vi "OSA_example.vi"() -> ()   [LabVIEW 2010]
doc: "Example GUI for continous or single asyncronous acquisition and plotting of interferogram and spectrum with datareduction. \n\nWhen creating custom dataacquisition applications displaying data; copy the graphs in this example, create corresponding graph references and connect to the init vi, see example diagram.\n\nRoutines with white icon background can be found in the TREE vi.\nRoutines with yellow icon background are specific for this example.\n\nMake sure there is no duplicate of FTSLV.dll, as otherwise FTSLib.dll and the Labview drivers might not be accessing the same library."
uses:
  _OSA_class/OSA.lvclass
  _OSA_class/typeDef/queue_action.ctl
  _OSA_class/typeDef/acq_dataType.ctl
  _OSA_class/typeDef/apodisation.ctl
  _OSA_class/misc_examples/ctrlRefs.ctl
  _OSA_class/misc_examples/action_data.ctl
  _OSA_class/typeDef/PDTemperatureMode.ctl
  _OSA_class/typeDef/resolution.ctl
  _OSA_class/typeDef/sensitivityMode.ctl
  _OSA_class/typeDef/spectrum_x_unit.ctl
  _OSA_class/misc_examples/y_unit_GUI.ctl
panel:
  in  "PD temp":T1
  in  "virtual OSA":bool=TRUE
  out "OSA":string="OSA20512 SN00001"
  out "status":string="STATUS OK "
  in  "acq delay (ms)":u32 step=200
  in  "resolution":T2
  in  "sensitivity":T3=enum."low medium"
  in  "ZOOM OUT BUTTON":bool
  in  "PANE RIGHT":bool
  in  "PANE LEFT":bool
  in  "cont acq butt":bool
  in  "ZOOM RESTORE":bool
  in  "ZOOM IN BUTTON":bool
  in  "exit butt":bool
  in  "single acq butt":bool
  in  "Tab Control":enum32{"interferogram", "spectrum"}(tab)=enum."spectrum"
  in  "gain":u16 max=100 step=1
  in  "auto":bool
  in  "wmtr":bool
  out "Wavemeter (/cm)":dbl format="%^.3e"
  out "Y intrfrgrm":T4={"X A intfgrm"=5, "X B intfrgrm"=52433, "X A-B intfrgrm"=52428} caption="Y"
  out "X intrfrgrm":T5={"X A intfgrm"=-0.008975722827017307, "X B intfrgrm"=-0.008905130438506603, "X A-B intfrgrm"=7.059238851070404e-05} caption="X" {"X A-B intfrgrm" format="%^.2e"; "X B intfrgrm" format="%.2f"; "X A intfgrm" format="%.2f"}
  in  "apodisation":T6
  out "Intensity Graph Interferogram":i32[][](graph)
  out "gain rel.":dbl=-1.0 format="%.1f"
  in  "coh.l":bool
  out "Coher.Length (cm)":dbl format="%^.3e"
  out "Signal (%)":dbl
  in  "Peak find":bool
  in  "pwr":bool
  out "Peak (X unit)":dbl format="%^.3e"
  out "Power (Y unit)":dbl format="%^.3e"
  out "X spectrum":T5={"X A intfgrm"=9482.365234375, "X B intfrgrm"=13082.42578125, "X A-B intfrgrm"=3600.060546875} caption="X" {"X A-B intfrgrm" format="%^.2e"; "X B intfrgrm" format="%.2f"; "X A intfgrm" format="%.2f"}
  out "Y spectrum":T5={"X A intfgrm"=0.0, "X B intfrgrm"=0.25791919231414795, "X A-B intfrgrm"=0.25791919231414795} caption="Y" {"X A-B intfrgrm" format="%^.2e"; "X B intfrgrm" format="%.2e"; "X A intfgrm" format="%.2e"}
  in  "rolling aver":bool
  in  "average nr":u16=1 min=1 max=100 step=1
  in  "spectrum x unit":T7
  in  "y unit":T8
  out "Intensity Graph spectrum":i32[][](graph)
  # "Right click to autoscale Y"
  # "Press scroll wheel for zoom in"
  # "Copy graphs if not building application from example."
  # "Copy graphs if not building application from example."
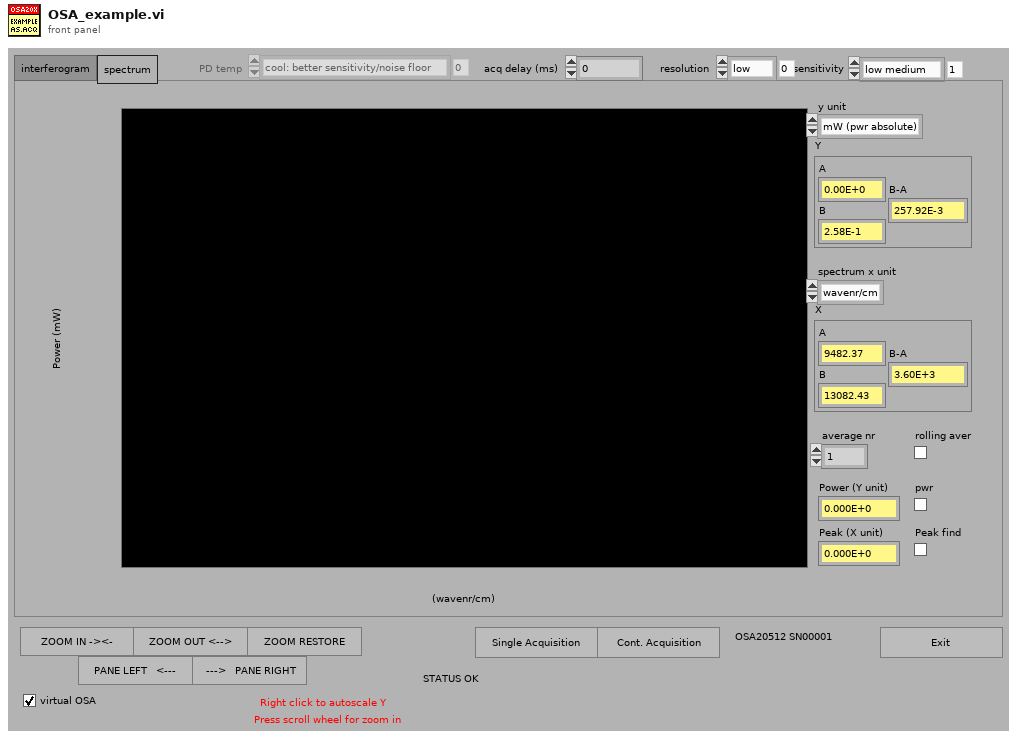
[diagram p1: front panel]
types:
  T1 = typedef "OSA.lvclass/PDTemperatureMode.ctl" = enum16{"cool: better sensitivity/noise floor", "warm: extended wl range"}
  T2 = typedef "OSA.lvclass/resolution.ctl" = enum16{"low", "high"}
  T3 = typedef "OSA.lvclass/sensitivityMode.ctl" = enum16{"low", "low medium", "high medium", "high"}
  T4 = cluster{"X A intfgrm":i32, "X B intfrgrm":i32, "X A-B intfrgrm":i32}
  T5 = cluster{"X A intfgrm":dbl, "X B intfrgrm":dbl, "X A-B intfrgrm":dbl}
  T6 = typedef "OSA.lvclass/apodisation.ctl" = enum16{"NONE", "NORTON_BEER_WEAK", "NORTON_BEER_MEDIUM", "NORTON_BEER_STRONG", "TRIANGULAR", "COSINE", "HANN", "HAMMING", "BLACKMANHARRIS3", "BLACKMANHARRIS4", "GAUSSIAN"}
  T7 = typedef "OSA.lvclass/spectrum_x_unit.ctl" = enum16{"wavenr/cm", "THz", "eV", "nm_air", "nm_vac"}
  T8 = typedef "OSA.lvclass/y_unit_GUI.ctl" = enum16{"mW (pwr absolute)", "dBm (pwr absolute)"}
  T9 = cluster{"waveCenter (nm)":dbl, "FWHM (nm)":dbl, "peakAmplitude":dbl}
  T10 = enum16{"OSA201", "OSA202", "OSA203", "OSA204", "OSA205", "OSA206", "OSA207", "OSA208"}
  T11 = typedef "OSA.lvclass/ctrlRefs.ctl" = cluster{"Peak (X unit)":refnum<vi>, "Power (Y unit)":refnum<vi>, "Wavemeter (/cm)":refnum<vi>, "Tab Control":refnum<vi>, "rolling average":refnum<vi>, "average nr":refnum<vi>, "apodisation":refnum<vi>, "acq delay (ms)":refnum<vi>, "sensitivity":refnum<vi>, "resolution":refnum<vi>, "WMtr":refnum<vi>, "X intrfrgrm":refnum<vi>, "Y intrfrgrm":refnum<vi>, "Y spectrum":refnum<vi>, "X spectrum":refnum<vi>, "single acq butt":refnum<vi>, "cont acq butt":refnum<vi>, "status ctrl":refnum<vi>, "auto":refnum<vi>, "gainLevel":refnum<vi>, "gain relative":refnum<vi>, "coh.L":refnum<vi>, "coherenceLength, (cm)":refnum<vi>, "Signal (%)":refnum<vi>, "PD mode":refnum<vi>, "wmtr":refnum<vi>, "pwr":refnum<vi>, "Peak find":refnum<vi>}
  T12 = typedef "OSA.lvclass/action_data.ctl" = cluster{"action":T13, "skip old":bool, "force immidiate":bool, "par":dbl, "par 2":dbl, "par 3":dbl, "par 4":dbl, "idx":i32, "idx 2":i32, "no duplicate":bool}
  T13 = typedef "OSA.lvclass/queue_action.ctl" = enum16{"none", "stop", "GUI_plotInterferogram", "GUI_plotSpectrum", "GUI_plotInterferogramRescale", "GUI_plotSpectrumRescale", "GUI_plotInterferogramReset", "GUI_plotSpectrumReset", "GUI_plotInterferogramAutoScaleY", "GUI_plotSpectrumAutoScaleY", "GUI_plotInterferogramZoomOut", "GUI_plotSpectrumZoomOut", "GUI_plotInterferogramPane", "GUI_plotSpectrumPane", "GUI_plotInterferogramZoomMouse", "GUI_plotSpectrumZoomMouse", "ENVIRONMENT temperature", "ENVIRONMENT pressure", "MODE_resolution set", "MODE_resolution get", "MODE_sensitivity set", "MODE_sensitivity get", "MODE_PDTemperature set", "MODE_PDTemperature get", "REBOOT/RESET firmware", "ACQASYNC_acquireSingleSpectrum", "ACQASYNC_continuous start", "ACQASYNC_continuous stop\n", "ACQASYNC_get last interferogram", "ACQASYNC_get last spectrum", "ACQASYNC_get last waveNr", "ACQOPT_interferogram smoothing set", "ACQOPT_interferogram smoothing get", "ACQOPT_spectrum smoothing set", "ACQOPT_spectrum smoothing get", "ACQOPT_apodisation type set", "ACQOPT_apodisation type get", "ACQOPT_phase correction type set", "ACQOPT_phase correction type get", "ACQOPT_acqIntervall_set", "ACQOPT_acqIntervall_get", "ACQOPT_average spectrum set", "ACQOPT_average spectrum get", "ACQOPT_rolling average set", "ACQOPT_rolling average get", "ACQOPT_zero fill factor set", "ACQOPT_zero fill factor get", "ACQOPT_cycle counting set", "ACQOPT_cycle counting get", "ACQOPT_air measure option set", "ACQOPT_air measure option get", "ACQOPT_gainLevel auto get", "ACQOPT_gainLevel auto set", "ACQOPT_gainLevel get", "ACQOPT_gainLevel set", "ACQOPT_getAll", "INSTRUMENT_PROPERTY_range_WaveNr_min", "INSTRUMENT_PROPERTY_range_WaveNr_max", "INSTRUMENT_PROPERTY_reference_wavelength_cm^-1", "INSTRUMENT_PROPERTY_samplesPerRefPeriod", "INSTRUMENT_PROPERTY_resolution_waveNrPercm", "INSTRUMENT_PROPERTY_availableGainLevels", "INSTRUMENT_PROPERTY_status", "CONVERT", "ANALYSE_POWER", "ANALYSE_PEAKS", "ANALYSE_WAVELENGTH", "ANALYSE_SPECTRUM", "ANALYSE_INTERFEROGRAM", "ANALYSE_COHERENCE_LENGTH", "MATH", "MATH_power", "MATH_peaks", "FILE", "miscellaneous"}
  T14 = typedef "OSA.lvclass/acq_dataType.ctl" = enum16{"none", "interferogram", "spectrum"}
  T15 = enum16{"pressure", "temperature", "humidity", "all"}
  T16 = typedef "LVPoint32TypeDef.ctl" = cluster{"Horizontal":i32, "Vertical":i32}
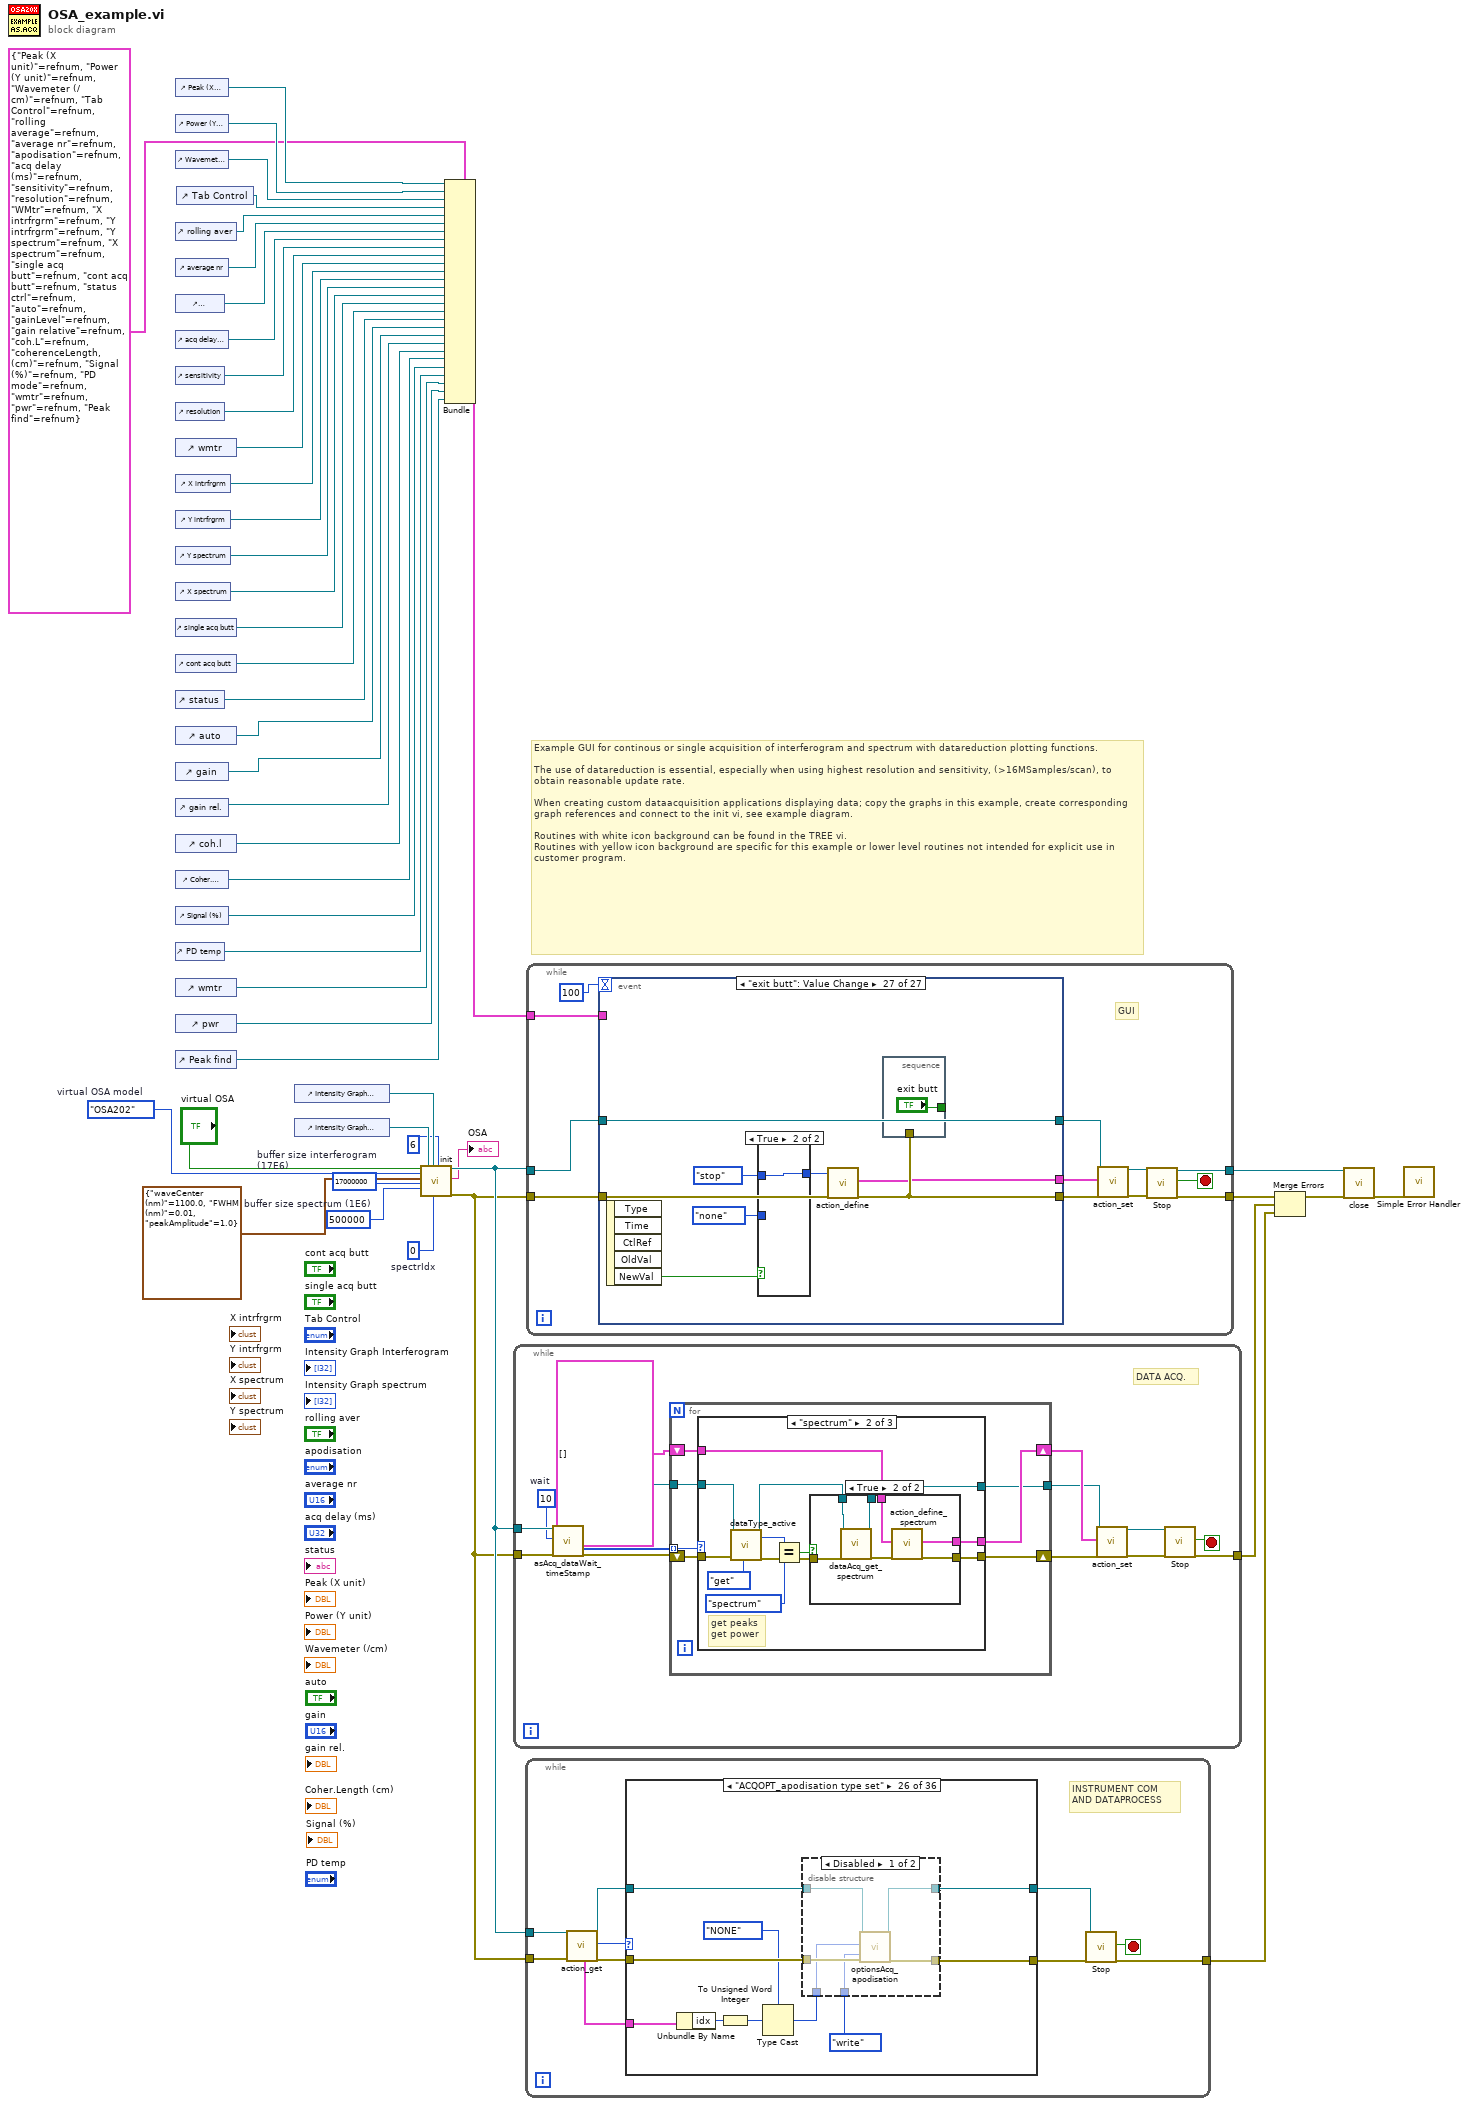
[diagram p0: block diagram]
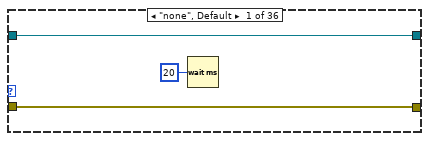
[diagram p2: hidden frame]
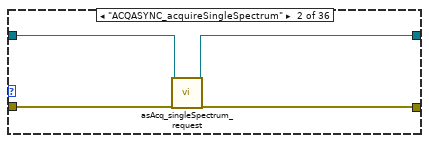
[diagram p3: hidden frame]
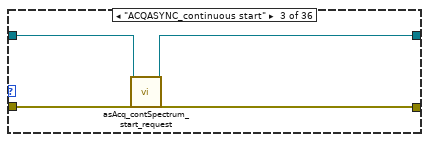
[diagram p4: hidden frame]
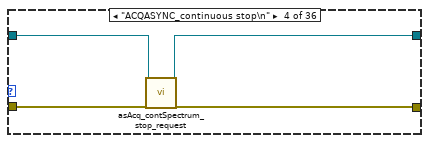
[diagram p5: hidden frame]
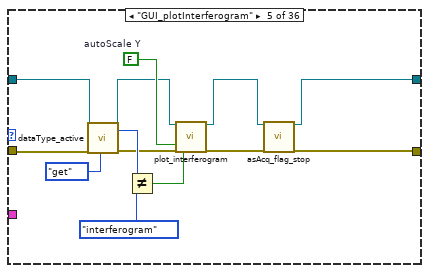
[diagram p6: hidden frame]
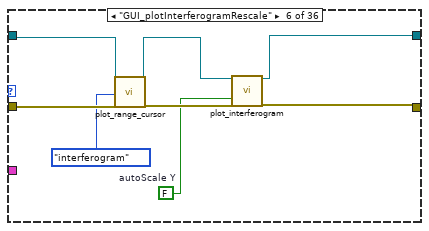
[diagram p7: hidden frame]
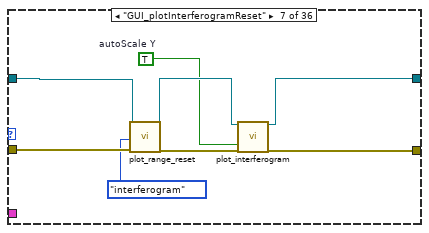
[diagram p8: hidden frame]
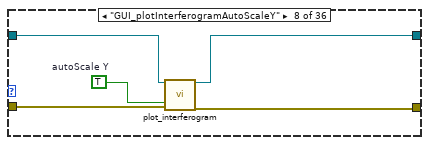
[diagram p9: hidden frame]
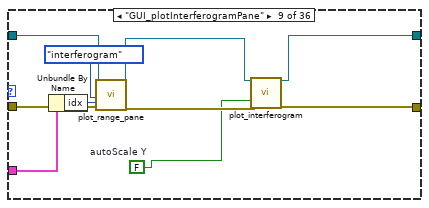
[diagram p10: hidden frame]
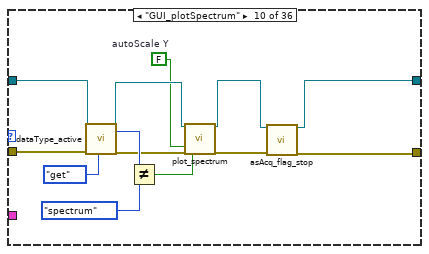
[diagram p11: hidden frame]
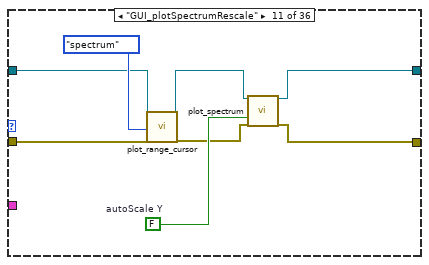
[diagram p12: hidden frame]
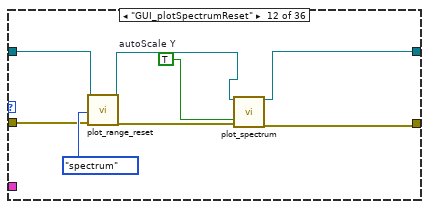
[diagram p13: hidden frame]
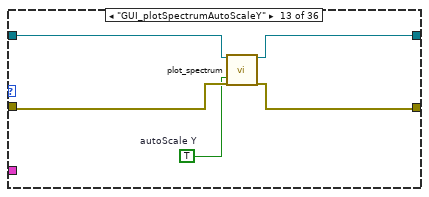
[diagram p14: hidden frame]
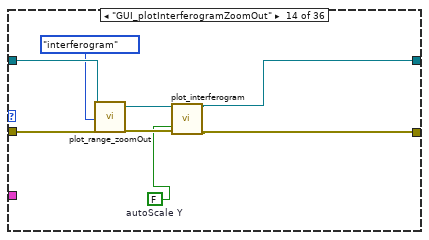
[diagram p15: hidden frame]
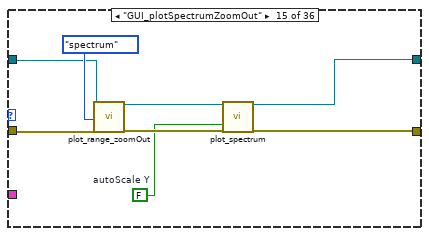
[diagram p16: hidden frame]
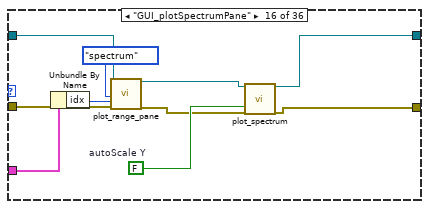
[diagram p17: hidden frame]
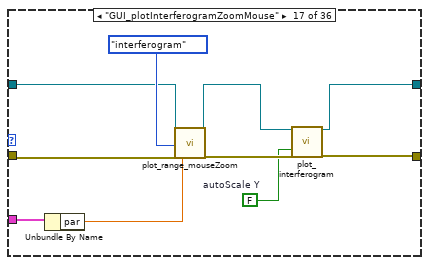
[diagram p18: hidden frame]
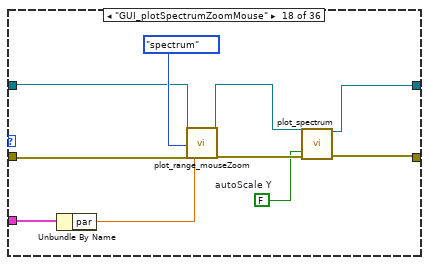
[diagram p19: hidden frame]
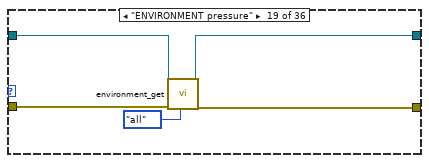
[diagram p20: hidden frame]
diagram:
  w5 = u16 0  # spectrIdx
  w8 = T10."OSA202"  # virtual OSA model
  w23 = 500000  # buffer size spectrum (1E6)
  w24 = 17000000  # buffer size interferogram (17E6)
  # "Example GUI for continous or single acquisition of interferogram and spectrum with datareduction plotting functions. \n\nThe use of datareduction is essential, especially when using highest resolution and sensitivity, (>16MSamples/scan), to obtain reasonable update rate.\n\nWhen creating custom dataacquisition applications displaying data; copy the graphs in this example, create corresponding graph references and connect to the init vi, see example diagram.\n\nRoutines with white icon background can be found in the TREE vi.\nRoutines with yellow icon background are specific for this example or lower level routines not intended for explicit use in customer program."
  n1 = control-ref of="Peak (X unit)"() -> (w27:refnum<vi>)
  n2 = control-ref of="Power (Y unit)"() -> (w28:refnum<vi>)
  n3 = control-ref of="Wavemeter (/cm)"() -> (w29:refnum<vi>)
  n4 = control-ref of="rolling aver"() -> (w42:refnum<vi>)
  n5 = control-ref of="average nr"() -> (w41:refnum<vi>)
  n6 = control-ref of="apodisation"() -> (w40:refnum<vi>)
  n7 = control-ref of="acq delay (ms)"() -> (w39:refnum<vi>)
  n8 = control-ref of="sensitivity"() -> (w38:refnum<vi>)
  n9 = control-ref of="resolution"() -> (w37:refnum<vi>)
  n10 = control-ref of="wmtr"() -> (w36:refnum<vi>)
  n11 = control-ref of="X intrfrgrm"() -> (w34:refnum<vi>)
  n12 = control-ref of="Y intrfrgrm"() -> (w33:refnum<vi>)
  n13 = control-ref of="Y spectrum"() -> (w32:refnum<vi>)
  n14 = control-ref of="X spectrum"() -> (w31:refnum<vi>)
  n15 = control-ref of="single acq butt"() -> (w22:refnum<vi>)
  n16 = control-ref of="cont acq butt"() -> (w21:refnum<vi>)
  n17 = control-ref of="status"() -> (w17:refnum<vi>)
  n18 = control-ref of="auto"() -> (w16:refnum<vi>)
  n19 = control-ref of="gain"() -> (w15:refnum<vi>)
  n20 = control-ref of="gain rel."() -> (w14:refnum<vi>)
  n21 = control-ref of="coh.l"() -> (w12:refnum<vi>)
  n22 = control-ref of="Coher.Length (cm)"() -> (w11:refnum<vi>)
  n23 = control-ref of="Signal (%)"() -> (w10:refnum<vi>)
  n24 = control-ref of="PD temp"() -> (w6:refnum<vi>)
  n25 = control-ref of="wmtr"() -> (w4:refnum<vi>)
  n26 = control-ref of="pwr"() -> (w3:refnum<vi>)
  n27 = control-ref of="Peak find"() -> (w2:refnum<vi>)
  n28 = control-ref of="Tab Control"() -> (w30:refnum<vi>)
  n29 = control-ref of="Intensity Graph spectrum"() -> (w43:refnum<vi>)
  n30 = control-ref of="Intensity Graph Interferogram"() -> (w44:refnum<vi>)
  n31 = call "init.vi"("virtual OSA"="virtual OSA", "virtual OSA model"=w8, "virtual OSA source"=T9 {"waveCenter (nm)"=1100.0, "FWHM (nm)"=0.01, "peakAmplitude"=1.0} ("source"), "buffer size interferogram (17E6)"=w24, "buffer size spectrum (1E6)"=w23, "Graph Intrfrgrm"=w44, "Graph Spectrum"=w43, "spectrIdx"=w5, 10:u16 6 ("channel (OSA300 only)")) -> ("duplicate reference"=w19:refnum<class "OSA.lvclass">, "spectrometer"=→"OSA":string, "error out"=w18:errorcluster)  [unwired: 6 in, 2 out]
  n32 = Bundle(cluster=T11 {"Peak (X unit)"=refnum, "Power (Y unit)"=refnum, "Wavemeter (/cm)"=refnum, "Tab Control"=refnum, "rolling average"=refnum, "average nr"=refnum, "apodisation"=refnum, "acq delay (ms)"=refnum, "sensitivity"=refnum, "resolution"=refnum, "WMtr"=refnum, "X intrfrgrm"=refnum, "Y intrfrgrm"=refnum, "Y spectrum"=refnum, "X spectrum"=refnum, "single acq butt"=refnum, "cont acq butt"=refnum, "status ctrl"=refnum, "auto"=refnum, "gainLevel"=refnum, "gain relative"=refnum, "coh.L"=refnum, "coherenceLength, (cm)"=refnum, "Signal (%)"=refnum, "PD mode"=refnum, "wmtr"=refnum, "pwr"=refnum, "Peak find"=refnum} ("ctrl refs"), "Peak (X unit)"=w27, "Power (Y unit)"=w28, "Wavemeter (/cm)"=w29, "Tab Control"=w30, "rolling average"=w42, "average nr"=w41, "apodisation"=w40, "acq delay (ms)"=w39, "sensitivity"=w38, "resolution"=w37, "WMtr"=w36, "X intrfrgrm"=w34, "Y intrfrgrm"=w33, "Y spectrum"=w32, "X spectrum"=w31, "single acq butt"=w22, "cont acq butt"=w21, "status ctrl"=w17, "auto"=w16, "gainLevel"=w15, "gain relative"=w14, "coh.L"=w12, "coherenceLength, (cm)"=w11, "Signal (%)"=w10, "PD mode"=w6, "wmtr"=w4, "pwr"=w3, "Peak find"=w2) -> (w35:T11)
  n33 = while {
    tunnel: w19 -> [w57]
    tunnel: w18 -> [w54]
    tunnel: [w62] -> w46
    stop <- w61 stop-if-true
    w53 = 10  # wait
    # "DATA ACQ."
    n34 = call "asAcq_dataWait_timeStamp.vi"("reference"=w57, "ms wait"=w53, "error in (no error)"=w54) -> ("duplicate reference"=w55:refnum<class "OSA.lvclass">, "dataType"=w52:T14[], "error out"=w56:errorcluster)  [unwired: 14 in]
    n35 = for {
      tunnel: w55 -> [w69]
      tunnel: [w63] -> w51
      shift-right: [w66] -> w50
      shift-left: w56 -> [w68]
      tunnel: w52 -> [w67] mode=indexing
      shift-right: [w65] -> w58
      shift-left: T12[] [] ("action data out") -> [w64]
      n36 = case shown="\"spectrum\"" w67 {
        tunnel: w68 -> [w80 w99 w114]
        tunnel: [w79 w93 w114] -> w66
        tunnel: w69 -> [w75 w97 w115]
        tunnel: [w78 w94 w115] -> w63
        tunnel: [w70 w92 w113] -> w65
        tunnel: w64 -> [w71 w91 w113]
        frame "interferogram", Default {
          n37 = call "dataType_active.vi"("reference"=w75, "get/set"=enum16{"get", "set"}."get") -> ("duplicate reference"=w73:refnum<class "OSA.lvclass">, "dataType active out"=w76:T14)  [unwired: 15 in, 1 out]
          n38 = Equal?(x=w76, y=acq_dataType."interferogram" ("dataType active out")) -> (x = y?=w74:bool)
          n39 = case shown="True" w74 {
            tunnel: w80 -> [w82 w87]
            tunnel: [w82 w90] -> w79
            tunnel: [w83 w84] -> w78
            tunnel: w73 -> [w83 w85]
            tunnel: w71 -> [w81 w89]
            tunnel: [w81 w88] -> w70
            frame False {
            }
            frame True {
              n40 = call-dynamic "dataAcq_get_interferogram.vi"("reference"=w85, "error in (no error)"=w87) -> ("duplicate reference"=w84:refnum<class "OSA.lvclass">, "error out"=w86:errorcluster)  [unwired: 16 in]
              n41 = call "action_define_interferogram.vi"("action data"=w89, "error in (no error)"=w86) -> ("action data out"=w88:T12[], "error out"=w90:errorcluster)  [unwired: 16 in]
            }
          }
        }
        frame "spectrum" {
          # "get peaks\nget power"
          n42 = call "dataType_active.vi"("reference"=w97, "error in (no error)"=w99, "get/set"=enum16{"get", "set"}."get") -> ("duplicate reference"=w98:refnum<class "OSA.lvclass">, "dataType active out"=w101:T14, "error out"=w96:errorcluster)  [unwired: 14 in]
          n43 = Equal?(x=w101, y=acq_dataType."spectrum" ("dataType active out")) -> (x = y?=w95:bool)
          n44 = case shown="True" w95 {
            tunnel: [w105 w109] -> w93
            tunnel: w98 -> [w104 w112]
            tunnel: w96 -> [w105 w111]
            tunnel: [w104 w106] -> w94
            tunnel: [w103 w108] -> w92
            tunnel: w91 -> [w103 w107]
            frame False {
            }
            frame True {
              n45 = call-dynamic "dataAcq_get_spectrum.vi"("reference"=w112, "error in (no error)"=w111) -> ("duplicate reference"=w106:refnum<class "OSA.lvclass">, "error out"=w110:errorcluster)  [unwired: 16 in]
              n46 = call "action_define_spectrum.vi"("action data"=w107, "error in (no error)"=w110) -> ("action data out"=w108:T12[], "error out"=w109:errorcluster)  [unwired: 16 in]
            }
          }
        }
        frame "none" {
        }
      }
    }
    n47 = call "action_set.vi"("reference"=w51, "action data"=w58, "error in (no error)"=w50) -> ("duplicate reference"=w59:refnum<class "OSA.lvclass">, "error out"=w60:errorcluster)  [unwired: 15 in]
    n48 = call "Stop.vi"("reference"=w59, "error in (no error)"=w60) -> ("Stop"=w61:bool, "error out"=w62:errorcluster)  [unwired: 15 in, 1 out]
  }
  n49 = while {
    tunnel: w19 -> [w120]
    tunnel: w18 -> [w123]
    tunnel: [w125] -> w45
    stop <- w124 stop-if-true
    # "INSTRUMENT COM\nAND DATAPROCESS"
    n50 = call "action_get.vi"("reference"=w120, "error in (no error)"=w123) -> ("action data"=w121:T12, "duplicate reference"=w119:refnum<class "OSA.lvclass">, "action"=w118:T13, "error out"=w122:errorcluster)  [unwired: 14 in]
    n51 = case shown="\"ACQOPT_apodisation type set\"" w118 {
      tunnel: [w128 w131 w135 w137 w143 w155 w165 w173 w178 w188 w200 w208 w216 w220 w230 w236 w250 w257 w269 w270 w278 w284 w290 w302 w304 w314 w332 w340 w343 w350 w364 w372 w376 w380 w385 w402] -> w117
      tunnel: w119 -> [w126 w129 w133 w139 w152 w160 w167 w171 w183 w197 w203 w211 w218 w225 w232 w242 w248 w260 w267 w273 w280 w286 w292 w301 w306 w316 w331 w339 w345 w356 w360 w371 w375 w379 w387 w408]
      tunnel: [w126 w130 w134 w138 w141 w157 w163 w172 w176 w186 w199 w207 w217 w221 w229 w237 w247 w258 w268 w271 w277 w285 w291 w300 w305 w315 w330 w338 w344 w351 w359 w370 w374 w378 w382 w403] -> w116
      tunnel: w122 -> [w128 w132 w136 w140 w153 w161 w169 w174 w184 w196 w204 w212 w215 w226 w233 w243 w249 w261 w266 w275 w281 w287 w289 w303 w307 w317 w333 w341 w349 w357 w365 w373 w377 w381 w388 w409]
      tunnel: w121 -> [_ _ _ _ _ _ _ _ w180 _ _ _ _ _ _ w240 w246 w262 _ w276 _ w288 _ w298 _ w311 w328 w336 w348 w354 w363 w369 _ _ _ _]
      frame "none", Default {
        n52 = Wait (ms)(milliseconds to wait=u32 20) -> ()  [unwired: 1 out]
      }
      frame "ACQASYNC_acquireSingleSpectrum" {
        n53 = call "asAcq_singleSpectrum_request.vi"("reference"=w129, "error in (no error)"=w132) -> ("duplicate reference"=w130:refnum<class "OSA.lvclass">, "error out"=w131:errorcluster)  [unwired: 16 in]
      }
      frame "ACQASYNC_continuous start" {
        n54 = call "asAcq_contSpectrum_start_request.vi"("reference"=w133, "error in (no error)"=w136) -> ("duplicate reference"=w134:refnum<class "OSA.lvclass">, "error out"=w135:errorcluster)  [unwired: 16 in]
      }
      frame "ACQASYNC_continuous stop\n" {
        n55 = call "asAcq_contSpectrum_stop_request.vi"("reference"=w139, "error in (no error)"=w140) -> ("duplicate reference"=w138:refnum<class "OSA.lvclass">, "error out"=w137:errorcluster)  [unwired: 16 in]
      }
      frame "GUI_plotInterferogram" {
        w146 = FALSE  # autoScale Y
        n56 = call "dataType_active.vi"("reference"=w152, "error in (no error)"=w153, "get/set"=enum16{"get", "set"}."get") -> ("duplicate reference"=w145:refnum<class "OSA.lvclass">, "dataType active out"=w150:T14, "error out"=w148:errorcluster)  [unwired: 14 in]
        n57 = Not Equal?(x=w150, y=acq_dataType."interferogram" ("dataType active out")) -> (x != y?=w147:bool)
        n58 = call "plot_interferogram.vi"("reference"=w145, "autoScale Y"=w146, "error in (no error)"=w148, "skip"=w147) -> ("duplicate reference"=w142:refnum<class "OSA.lvclass">, "error out"=w144:errorcluster)  [unwired: 14 in]
        n59 = call "asAcq_flag_stop.vi"("reference"=w142, "error in (no error)"=w144) -> ("duplicate reference"=w141:refnum<class "OSA.lvclass">, "error out"=w143:errorcluster)  [unwired: 16 in]
      }
      frame "GUI_plotInterferogramRescale" {
        w154 = FALSE  # autoScale Y
        n60 = call "plot_range_cursor.vi"("reference"=w160, "dataType"=acq_dataType."interferogram", "error in (no error)"=w161) -> ("duplicate reference"=w158:refnum<class "OSA.lvclass">, "error out"=w156:errorcluster)  [unwired: 15 in]
        n61 = call "plot_interferogram.vi"("reference"=w158, "autoScale Y"=w154, "error in (no error)"=w156) -> ("duplicate reference"=w157:refnum<class "OSA.lvclass">, "error out"=w155:errorcluster)  [unwired: 15 in]
      }
      frame "GUI_plotInterferogramReset" {
        w162 = TRUE  # autoScale Y
        n62 = call "plot_range_reset.vi"("reference"=w167, "dataType"=acq_dataType."interferogram", "error in (no error)"=w169) -> ("duplicate reference"=w164:refnum<class "OSA.lvclass">, "error out"=w166:errorcluster)  [unwired: 15 in]
        n63 = call "plot_interferogram.vi"("reference"=w164, "autoScale Y"=w162, "error in (no error)"=w166) -> ("duplicate reference"=w163:refnum<class "OSA.lvclass">, "error out"=w165:errorcluster)  [unwired: 15 in]
      }
      frame "GUI_plotInterferogramAutoScaleY" {
        w170 = TRUE  # autoScale Y
        n64 = call "plot_interferogram.vi"("reference"=w171, "autoScale Y"=w170, "error in (no error)"=w174) -> ("duplicate reference"=w172:refnum<class "OSA.lvclass">, "error out"=w173:errorcluster)  [unwired: 15 in]
      }
      frame "GUI_plotInterferogramPane" {
        w175 = FALSE  # autoScale Y
        n65 = Unbundle By Name(w180) -> ("idx"=w182:i32)
        n66 = call "plot_range_pane.vi"("reference"=w183, "dataType"=acq_dataType."interferogram", "direction"=w182, "error in (no error)"=w184) -> ("duplicate reference"=w177:refnum<class "OSA.lvclass">, "error out"=w179:errorcluster)  [unwired: 14 in]
        n67 = call "plot_interferogram.vi"("reference"=w177, "autoScale Y"=w175, "error in (no error)"=w179) -> ("duplicate reference"=w176:refnum<class "OSA.lvclass">, "error out"=w178:errorcluster)  [unwired: 15 in]
      }
      frame "GUI_plotSpectrum" {
        w190 = FALSE  # autoScale Y
        n68 = call "dataType_active.vi"("reference"=w197, "error in (no error)"=w196, "get/set"=enum16{"get", "set"}."get") -> ("duplicate reference"=w191:refnum<class "OSA.lvclass">, "dataType active out"=w194:T14, "error out"=w192:errorcluster)  [unwired: 14 in]
        n69 = Not Equal?(x=w194, y=acq_dataType."spectrum" ("dataType active out")) -> (x != y?=w185:bool)
        n70 = call "plot_spectrum.vi"("reference"=w191, "autoScale Y"=w190, "error in (no error)"=w192, "skip"=w185) -> ("duplicate reference"=w187:refnum<class "OSA.lvclass">, "error out"=w189:errorcluster)  [unwired: 14 in]
        n71 = call "asAcq_flag_stop.vi"("reference"=w187, "error in (no error)"=w189) -> ("duplicate reference"=w186:refnum<class "OSA.lvclass">, "error out"=w188:errorcluster)  [unwired: 16 in]
      }
      frame "GUI_plotSpectrumRescale" {
        w202 = FALSE  # autoScale Y
        n72 = call "plot_range_cursor.vi"("reference"=w203, "dataType"=acq_dataType."spectrum", "error in (no error)"=w204) -> ("duplicate reference"=w198:refnum<class "OSA.lvclass">, "error out"=w201:errorcluster)  [unwired: 15 in]
        n73 = call "plot_spectrum.vi"("reference"=w198, "autoScale Y"=w202, "error in (no error)"=w201) -> ("duplicate reference"=w199:refnum<class "OSA.lvclass">, "error out"=w200:errorcluster)  [unwired: 15 in]
      }
      frame "GUI_plotSpectrumReset" {
        w210 = TRUE  # autoScale Y
        n74 = call "plot_range_reset.vi"("reference"=w211, "dataType"=acq_dataType."spectrum", "error in (no error)"=w212) -> ("duplicate reference"=w206:refnum<class "OSA.lvclass">, "error out"=w209:errorcluster)  [unwired: 15 in]
        n75 = call "plot_spectrum.vi"("reference"=w206, "autoScale Y"=w210, "error in (no error)"=w209) -> ("duplicate reference"=w207:refnum<class "OSA.lvclass">, "error out"=w208:errorcluster)  [unwired: 15 in]
      }
      frame "GUI_plotSpectrumAutoScaleY" {
        w214 = TRUE  # autoScale Y
        n76 = call "plot_spectrum.vi"("reference"=w218, "autoScale Y"=w214, "error in (no error)"=w215) -> ("duplicate reference"=w217:refnum<class "OSA.lvclass">, "error out"=w216:errorcluster)  [unwired: 15 in]
      }
      frame "GUI_plotInterferogramZoomOut" {
        w219 = FALSE  # autoScale Y
        n77 = call "plot_range_zoomOut.vi"("reference"=w225, "dataType"=acq_dataType."interferogram", "error in (no error)"=w226) -> ("duplicate reference"=w222:refnum<class "OSA.lvclass">, "error out"=w223:errorcluster)  [unwired: 15 in]
        n78 = call "plot_interferogram.vi"("reference"=w222, "autoScale Y"=w219, "error in (no error)"=w223) -> ("duplicate reference"=w221:refnum<class "OSA.lvclass">, "error out"=w220:errorcluster)  [unwired: 15 in]
      }
      frame "GUI_plotSpectrumZoomOut" {
        w227 = FALSE  # autoScale Y
        n79 = call "plot_range_zoomOut.vi"("reference"=w232, "dataType"=acq_dataType."spectrum", "error in (no error)"=w233) -> ("duplicate reference"=w228:refnum<class "OSA.lvclass">, "error out"=w231:errorcluster)  [unwired: 15 in]
        n80 = call "plot_spectrum.vi"("reference"=w228, "autoScale Y"=w227, "error in (no error)"=w231) -> ("duplicate reference"=w229:refnum<class "OSA.lvclass">, "error out"=w230:errorcluster)  [unwired: 15 in]
      }
      frame "GUI_plotSpectrumPane" {
        w239 = FALSE  # autoScale Y
        n81 = Unbundle By Name(w240) -> ("idx"=w241:i32)
        n82 = call "plot_range_pane.vi"("reference"=w242, "dataType"=acq_dataType."spectrum", "direction"=w241, "error in (no error)"=w243) -> ("duplicate reference"=w238:refnum<class "OSA.lvclass">, "error out"=w235:errorcluster)  [unwired: 14 in]
        n83 = call "plot_spectrum.vi"("reference"=w238, "autoScale Y"=w239, "error in (no error)"=w235) -> ("duplicate reference"=w237:refnum<class "OSA.lvclass">, "error out"=w236:errorcluster)  [unwired: 15 in]
      }
      frame "GUI_plotInterferogramZoomMouse" {
        w251 = FALSE  # autoScale Y
        n84 = Unbundle By Name(w246) -> ("par"=w245:dbl)
        n85 = call "plot_range_mouseZoom.vi"("reference"=w248, "dataType"=acq_dataType."interferogram", "error in (no error)"=w249, "X mouse"=w245) -> ("duplicate reference"=w253:refnum<class "OSA.lvclass">, "error out"=w252:errorcluster)  [unwired: 14 in]
        n86 = call "plot_interferogram.vi"("reference"=w253, "autoScale Y"=w251, "error in (no error)"=w252) -> ("duplicate reference"=w247:refnum<class "OSA.lvclass">, "error out"=w250:errorcluster)  [unwired: 15 in]
      }
      frame "GUI_plotSpectrumZoomMouse" {
        w255 = FALSE  # autoScale Y
        n87 = Unbundle By Name(w262) -> ("par"=w263:dbl)
        n88 = call "plot_range_mouseZoom.vi"("reference"=w260, "dataType"=acq_dataType."spectrum", "error in (no error)"=w261, "X mouse"=w263) -> ("duplicate reference"=w259:refnum<class "OSA.lvclass">, "error out"=w256:errorcluster)  [unwired: 14 in]
        n89 = call "plot_spectrum.vi"("reference"=w259, "autoScale Y"=w255, "error in (no error)"=w256) -> ("duplicate reference"=w258:refnum<class "OSA.lvclass">, "error out"=w257:errorcluster)  [unwired: 15 in]
      }
      frame "ENVIRONMENT pressure" {
        n90 = call "environment_get.vi"("reference"=w267, "error in (no error)"=w266, "parameter"=T15."all") -> ("duplicate reference"=w268:refnum<class "OSA.lvclass">, "error out"=w269:errorcluster)  [unwired: 9 in, 6 out]
      }
      frame "MODE_resolution set" {
        n91 = Unbundle By Name(w276) -> ("idx"=w274:i32)
        n92 = call "mode_resolution.vi"("reference"=w273, "resolution"=w274, "error in (no error)"=w275, "read/write"=enum16{"read", "write"}."write") -> ("duplicate reference"=w271:refnum<class "OSA.lvclass">, "error out"=w270:errorcluster)  [unwired: 12 in, 2 out]
      }
      frame "MODE_resolution get" {
        n93 = call "mode_resolution.vi"("reference"=w280, "error in (no error)"=w281, "read/write"=enum16{"read", "write"}."read") -> ("duplicate reference"=w277:refnum<class "OSA.lvclass">, "error out"=w278:errorcluster)  [unwired: 13 in, 2 out]
      }
      frame "MODE_sensitivity set" {
        n94 = Unbundle By Name(w288) -> ("idx"=w283:i32)
        n95 = call "mode_sensitivity.vi"("reference"=w286, "sensitivity"=w283, "error in (no error)"=w287, "read/write"=enum16{"read", "write"}."write") -> ("duplicate reference"=w285:refnum<class "OSA.lvclass">, "error out"=w284:errorcluster)  [unwired: 13 in, 1 out]
      }
      frame "MODE_sensitivity get" {
        n96 = call "mode_sensitivity.vi"("reference"=w292, "error in (no error)"=w289, "read/write"=enum16{"read", "write"}."read") -> ("duplicate reference"=w291:refnum<class "OSA.lvclass">, "error out"=w290:errorcluster)  [unwired: 14 in, 1 out]
      }
      frame "MODE_PDTemperature set" {
        n97 = Unbundle By Name(w298) -> ("idx"=w297:i32)
        n98 = To Unsigned Word Integer(number=w297) -> (unsigned 16bit integer=w296:u16)
        n99 = Type Cast(type=PDTemperatureMode."cool: better sensitivity/noise floor" ("PD sensitivity mode"), x=w296) -> (*(type *) &x=w294:T1)
        n100 = call "optionsAcq_PDTemperatureMode.vi"("reference"=w301, "PD sensitivity mode"=w294, "error in (no error)"=w303, "read/write"=enum16{"read", "write"}."write") -> ("duplicate reference"=w300:refnum<class "OSA.lvclass">, "error out"=w302:errorcluster)  [unwired: 12 in, 2 out]
      }
      frame "ACQOPT_getAll" {
        n101 = call "optionsAcq_getAll.vi"("reference"=w306, "error in (no error)"=w307) -> ("duplicate reference"=w305:refnum<class "OSA.lvclass">, "error out"=w304:errorcluster)  [unwired: 10 in, 14 out]
      }
      frame "ACQOPT_apodisation type set" {
        n102 = Unbundle By Name(w311) -> ("idx"=w310:i32)
        n103 = To Unsigned Word Integer(number=w310) -> (unsigned 16bit integer=w308:u16)
        n104 = Type Cast(type=apodisation."NONE" ("apodisation"), x=w308) -> (*(type *) &x=w309:T6)
        n105 = disable-structure shown="Disabled" {
          disable-tunnel: w317 -> [w323 w324]
          disable-tunnel: w316 -> [w322 w325]
          disable-tunnel: [w321 w325] -> w315
          disable-tunnel: [w320 w324] -> w314
          disable-tunnel: enum16{"read", "write"}."write" ("readWrite") -> [w319 _]
          disable-tunnel: w309 -> [w318 _]
          frame Disabled {
            n106 = call "optionsAcq_apodisation.vi"("reference"=w322, "apodisation"=w318, "readWrite"=w319, "error in (no error)"=w323) -> ("duplicate reference"=w321:refnum<class "OSA.lvclass">, "error out"=w320:errorcluster)  [unwired: 12 in, 2 out]
          }
          frame Enabled {
          }
        }
      }
      frame "ACQOPT_rolling average set" {
        n107 = Unbundle By Name(w328) -> ("idx"=w327:i32)
        n108 = Greater Than 0?(x=w327) -> (x > 0?=w326:bool)
        n109 = call "optionsAcq_average_rolling.vi"("reference"=w331, "rolling"=w326, "readWrite"=enum16{"read", "write"}."write", "error in (no error)"=w333) -> ("duplicate reference"=w330:refnum<class "OSA.lvclass">, "error out"=w332:errorcluster)  [unwired: 12 in, 2 out]
      }
      frame "ACQOPT_average spectrum set" {
        n110 = Unbundle By Name(w336) -> ("idx"=w335:i32)
        n111 = To Unsigned Long Integer(number=w335) -> (unsigned 32bit integer=w334:u32)
        n112 = call "optionsAcq_averageSpectrum.vi"("reference"=w339, "average"=w334, "readWrite"=enum16{"read", "write"}."write", "error in (no error)"=w341) -> ("duplicate reference"=w338:refnum<class "OSA.lvclass">, "error out"=w340:errorcluster)  [unwired: 12 in, 2 out]
      }
      frame "ACQOPT_acqIntervall_set" {
        n113 = Unbundle By Name(w348) -> ("idx"=w347:i32)
        n114 = To Unsigned Long Integer(number=w347) -> (unsigned 32bit integer=w346:u32)
        n115 = call "optionsAcq_acqRate.vi"("reference"=w345, "intervall (ms)"=w346, "readWrite"=enum16{"read", "write"}."write", "error in (no error)"=w349) -> ("duplicate reference"=w344:refnum<class "OSA.lvclass">, "error out"=w343:errorcluster)  [unwired: 13 in, 1 out]
      }
      frame "ACQOPT_cycle counting set" {
        n116 = Unbundle By Name(w354) -> ("idx"=w353:i32)
        n117 = Greater Than 0?(x=w353) -> (x > 0?=w352:bool)
        n118 = call-dynamic "optionsAcq_cycleCountingWavemeter.vi"("reference"=w356, "cycleCounting"=w352, "readWrite"=enum16{"read", "write"}."write", "error in (no error)"=w357) -> ("duplicate reference"=w351:refnum<class "OSA.lvclass">, "error out"=w350:errorcluster)  [unwired: 12 in, 2 out]
      }
      frame "ACQOPT_gainLevel auto set" {
        n119 = Unbundle By Name(w363) -> ("idx"=w362:i32)
        n120 = Greater Than 0?(x=w362) -> (x > 0?=w361:bool)
        n121 = call-dynamic "optionsAcq_gainAuto.vi"("reference"=w360, "auto"=w361, "readWrite"=enum16{"read", "write"}."write", "error in (no error)"=w365) -> ("duplicate reference"=w359:refnum<class "OSA.lvclass">, "error out"=w364:errorcluster)  [unwired: 12 in, 2 out]
      }
      frame "ACQOPT_gainLevel set" {
        n122 = Unbundle By Name(w369) -> ("idx"=w368:i32)
        n123 = To Unsigned Word Integer(number=w368) -> (unsigned 16bit integer=w367:u16)
        n124 = call "optionsAcq_gainOpticalDetector.vi"("reference"=w371, "gain_idx"=w367, "readWrite"=enum16{"read", "write"}."write", "error in (no error)"=w373) -> ("duplicate reference"=w370:refnum<class "OSA.lvclass">, "error out"=w372:errorcluster)  [unwired: 11 in, 3 out]
      }
      frame "INSTRUMENT_PROPERTY_resolution_waveNrPercm" {
        n125 = call "instrumentProperties_resolution_WaveNr.vi"("reference"=w375, "error in (no error)"=w377) -> ("duplicate reference"=w374:refnum<class "OSA.lvclass">, "error out"=w376:errorcluster)  [unwired: 15 in, 1 out]
      }
      frame "INSTRUMENT_PROPERTY_status" {
        n126 = call "instrumentProperties_status.vi"("reference"=w379, "error in (no error)"=w381) -> ("duplicate reference"=w378:refnum<class "OSA.lvclass">, "error out"=w380:errorcluster)  [unwired: 12 in, 4 out]
      }
      frame "ANALYSE_SPECTRUM" {
        # "calc power\ncalc peaks"
        n127 = case shown="True" "Peak find" {
          tunnel: w388 -> [w396 w401]
          tunnel: w387 -> [w397 w399]
          tunnel: [w396 w400] -> w386
          tunnel: [w397 w398] -> w383
          frame False {
          }
          frame True {
            n128 = call "peak_find.vi"("reference"=w399, "error in (no error)"=w401) -> ("reference out"=w398:refnum<class "OSA.lvclass">, "error out"=w400:errorcluster)  [unwired: 16 in]
          }
        }
        n129 = case shown="True" "pwr" {
          tunnel: w386 -> [w390 w393]
          tunnel: [w390 w392] -> w385
          tunnel: w383 -> [w391 w395]
          tunnel: [w391 w394] -> w382
          frame False {
          }
          frame True {
            n130 = call "power_get.vi"("reference"=w395, "error in (no error)"=w393) -> ("reference out"=w394:refnum<class "OSA.lvclass">, "error out"=w392:errorcluster)  [unwired: 16 in]
          }
        }
      }
      frame "ANALYSE_INTERFEROGRAM" {
        n131 = case shown="True" "wmtr" {
          tunnel: w409 -> [w416 w421]
          tunnel: w408 -> [w417 w420]
          tunnel: [w417 w419] -> w405
          tunnel: [w416 w418] -> w406
          frame False {
          }
          frame True {
            n132 = call "dataAcq_get_wavelengthMeter.vi"("reference"=w420, "error in (no error)"=w421) -> ("duplicate reference"=w419:refnum<class "OSA.lvclass">, "error out"=w418:errorcluster)  [unwired: 15 in, 1 out]
          }
        }
        n133 = case shown="True" "coh.l" {
          tunnel: w406 -> [w410 w415]
          tunnel: w405 -> [w411 w413]
          tunnel: [w411 w412] -> w403
          tunnel: [w410 w414] -> w402
          frame False {
          }
          frame True {
            n134 = call "dataProcess_coherenceLength.vi"("reference"=w413, "error in (no error)"=w415) -> ("duplicate reference"=w412:refnum<class "OSA.lvclass">, "error out"=w414:errorcluster)  [unwired: 14 in, 2 out]
          }
        }
      }
    }
    n135 = call "Stop.vi"("reference"=w116, "error in (no error)"=w117) -> ("Stop"=w124:bool, "error out"=w125:errorcluster)  [unwired: 15 in, 1 out]
  }
  n136 = while {
    tunnel: w18 -> [w433]
    tunnel: [w432] -> w47
    tunnel: w19 -> [w431]
    tunnel: [w430] -> w25
    tunnel: w35 -> [w422]
    stop <- w429 stop-if-true
    # "GUI"
    n137 = event shown="[26] \"exit butt\": Value Change" {
      selector: _ -> [_ _ _ _ _ _ _ _ _ _ _ _ _ _ _ _ _ _ _ _ _ _ _ _ _ _ _]
      dyn-events: _ -> [_ _ _ _ _ _ _ _ _ _ _ _ _ _ _ _ _ _ _ _ _ _ _ _ _ _ _]
      timeout: 100 -> [_ _ _ _ _ _ _ _ _ _ _ _ _ _ _ _ _ _ _ _ _ _ _ _ _ _ _]
      tunnel: w433 -> [w446 w456 w465 w477 w488 w503 w522 w529 w565 w589 w597 w608 w615 w624 w633 w645 w655 w660 w665 w671 w689 w712 w723 w743 w754 w764 w772]
      tunnel: [w438 w464 w472 w474 w484 w498 w517 w543 w564 w590 w599 w610 w614 w627 w634 w643 w654 w659 w664 w677 w692 w704 w719 w742 w753 w763 w771] -> w427
      tunnel: w431 -> [w449 w461 w467 w476 w487 w501 w521 w544 w562 w592 w596 w604 w612 w623 w632 w642 w647 w657 w662 w675 w693 w711 w725 w737 w745 w758 w769]
      tunnel: [w442 w461 w467 w478 w486 w494 w520 w544 w562 w592 w596 w604 w612 w623 w632 w642 w647 w657 w662 w675 w693 w711 w725 w737 w745 w758 w769] -> w426
      tunnel: [w440 w463 w471 w479 w489 w497 w519 w531 w563 w591 w598 w609 w613 w626 w631 w644 w653 w658 w663 w676 w691 w705 w722 w741 w746 w759 w770] -> w423
      tunnel: w422 -> [w444 _ _ _ _ _ _ _ _ _ _ _ _ _ _ _ _ _ _ w669 w688 w709 w721 _ w756 _ _]
      event Timeout {
        n138 = event-data() -> ()  [unwired: 1 in, 1 out]
        n139 = call "GUI_update.vi"("reference"=w449, "error in (no error)"=w446, "ctrl refs"=w444, "y unit"="y unit", "spectrum x unit"="spectrum x unit") -> ("acq stopped"=w437:bool, "duplicate reference"=w443:refnum<class "OSA.lvclass">, "error out"=w445:errorcluster)  [unwired: 8 in, 4 out]
        n140 = call "GUI_optionsUpdate.vi"("reference"=w443, "error in (no error)"=w445, "ctrl refs"=w444) -> ("duplicate reference"=w442:refnum<class "OSA.lvclass">, "error out"=w439:errorcluster)  [unwired: 15 in]
        n141 = Select(t=T13[] [enum."INSTRUMENT_PROPERTY_status", enum."ACQOPT_getAll", enum."MODE_resolution get", enum."MODE_sensitivity get"], s=w437, f=T13[] [enum."INSTRUMENT_PROPERTY_status", enum."MODE_resolution get", enum."MODE_sensitivity get"]) -> (s? t:f=w434:T13[])
        n142 = for {
          shift-right: [w454] -> w440
          shift-left: T12[] [] ("action data out") -> [w452]
          tunnel: w434 -> [w453] mode=indexing
          shift-right: [w451] -> w438
          shift-left: w439 -> [w450]
          w455 = TRUE  # skip old
          n143 = call "action_define.vi"("action"=w453, "action data"=w452, "error in (no error)"=w450, "skip old"=w455) -> ("action data out"=w454:T12[], "error out"=w451:errorcluster)  [unwired: 14 in]
        }
      }
      event "single acq butt": Value Change {
        w462 = TRUE  # skip old
        n144 = event-data() -> ("NewVal"=w460:bool)  [unwired: 1 in, 4 out]
        n145 = Select(t=queue_action."ACQASYNC_acquireSingleSpectrum" ("action"), s=w460, f=queue_action."none" ("action")) -> (s? t:f=w457:T13)
        n146 = call "action_define.vi"("action"=w457, "error in (no error)"=w456, "skip old"=w462) -> ("action data out"=w463:T12[], "error out"=w464:errorcluster)  [unwired: 15 in]
      }
      event "cont acq butt": Value Change {
        w473 = TRUE  # skip old
        n147 = event-data() -> ("NewVal"=w466:bool)  [unwired: 1 in, 4 out]
        n148 = Select(t=queue_action."ACQASYNC_continuous start" ("action"), s=w466, f=queue_action."ACQASYNC_continuous stop\n" ("action")) -> (s? t:f=w468:T13)
        n149 = call "action_define.vi"("action"=w468, "error in (no error)"=w465, "skip old"=w473) -> ("action data out"=w471:T12[], "error out"=w472:errorcluster)  [unwired: 15 in]
      }
      event "ZOOM IN BUTTON": Value Change {
        w480 = cluster{"action":T13, "skip old":bool}[] [{"action"=enum."GUI_plotInterferogramRescale", "skip old"=FALSE}, {"action"=enum."ANALYSE_INTERFEROGRAM", "skip old"=TRUE}]  # action interferogram
        w481 = cluster{"action":T13, "skip old":bool}[] [{"action"=enum."GUI_plotSpectrumRescale", "skip old"=FALSE}, {"action"=enum."ANALYSE_SPECTRUM", "skip old"=TRUE}]  # action spectrum
        n150 = event-data() -> ()  [unwired: 1 in, 5 out]
        n151 = call "GUILoop_plotUpdate_cmds.vi"("reference"=w476, "error in (no error)"=w477, "action interferogram"=w480, "action spectrum"=w481) -> ("reference out"=w478:refnum<class "OSA.lvclass">, "action data out"=w479:T12[], "error out"=w475:errorcluster)  [unwired: 13 in]
        n152 = stacked-sequence {
          tunnel: w475 -> [w483]
          tunnel: [w483] -> w474
          tunnel: ["ZOOM IN BUTTON"] -> _
          frame #0 {
          }
        }
      }
      event "ZOOM OUT BUTTON": Value Change {
        w490 = cluster{"action":T13, "skip old":bool}[] [{"action"=enum."GUI_plotSpectrumZoomOut", "skip old"=FALSE}, {"action"=enum."ANALYSE_SPECTRUM", "skip old"=TRUE}]  # action spectrum
        w491 = cluster{"action":T13, "skip old":bool}[] [{"action"=enum."GUI_plotInterferogramZoomOut", "skip old"=FALSE}, {"action"=enum."ANALYSE_INTERFEROGRAM", "skip old"=TRUE}]  # action interferogram
        n153 = event-data() -> ()  [unwired: 1 in, 5 out]
        n154 = call "GUILoop_plotUpdate_cmds.vi"("reference"=w487, "error in (no error)"=w488, "action interferogram"=w491, "action spectrum"=w490) -> ("reference out"=w486:refnum<class "OSA.lvclass">, "action data out"=w489:T12[], "error out"=w485:errorcluster)  [unwired: 13 in]
        n155 = stacked-sequence {
          tunnel: w485 -> [w492]
          tunnel: ["ZOOM OUT BUTTON"] -> _
          tunnel: [w492] -> w484
          frame #0 {
          }
        }
      }
      event "PANE RIGHT", "PANE LEFT": Value Change {
        n156 = event-data() -> ()  [unwired: 1 in, 5 out]
        n157 = call "dataType_active.vi"("reference"=w501, "error in (no error)"=w503, "get/set"=enum16{"get", "set"}."get") -> ("duplicate reference"=w494:refnum<class "OSA.lvclass">, "dataType active out"=w500:T14, "error out"=w502:errorcluster)  [unwired: 14 in]
        n158 = Build Array("PANE LEFT", "PANE RIGHT") -> (w510:bool[])
        n159 = case shown="\"interferogram\", Default" w500 {
          tunnel: queue_action."GUI_plotSpectrumPane" ("action") -> [_ w516]
          tunnel: queue_action."GUI_plotInterferogramPane" ("action") -> [w514 _]
          tunnel: [w514 w516] -> w505
          tunnel: [queue_action."ANALYSE_INTERFEROGRAM" ("action") queue_action."ANALYSE_SPECTRUM" ("action")] -> w495
          frame "interferogram", Default {
          }
          frame "spectrum" {
          }
        }
        n160 = Search 1D Array(1D array=w510, element=TRUE) -> (index of element=w508:i32)  [unwired: 1 in]
        n161 = call "action_define.vi"("action"=w505, "error in (no error)"=w502, "idx"=w508) -> ("action data out"=w496:T12[], "error out"=w499:errorcluster)  [unwired: 15 in]
        n162 = call "action_define.vi"("action"=w495, "action data"=w496, "error in (no error)"=w499) -> ("action data out"=w497:T12[], "error out"=w498:errorcluster)  [unwired: 15 in]
      }
      event "ZOOM RESTORE": Value Change {
        w523 = cluster{"action":T13, "skip old":bool}[] [{"action"=enum."GUI_plotInterferogramReset", "skip old"=FALSE}, {"action"=enum."ANALYSE_INTERFEROGRAM", "skip old"=TRUE}]  # action interferogram
        w524 = cluster{"action":T13, "skip old":bool}[] [{"action"=enum."GUI_plotSpectrumReset", "skip old"=FALSE}, {"action"=enum."ANALYSE_SPECTRUM", "skip old"=TRUE}]  # action spectrum
        n163 = event-data() -> ()  [unwired: 1 in, 5 out]
        n164 = call "GUILoop_plotUpdate_cmds.vi"("reference"=w521, "error in (no error)"=w522, "action interferogram"=w523, "action spectrum"=w524) -> ("reference out"=w520:refnum<class "OSA.lvclass">, "action data out"=w519:T12[], "error out"=w518:errorcluster)  [unwired: 13 in]
        n165 = stacked-sequence {
          tunnel: w518 -> [w525]
          tunnel: ["ZOOM RESTORE"] -> _
          tunnel: [w525] -> w517
          frame #0 {
          }
        }
      }
      event "Intensity Graph spectrum": Mouse Up {
        n166 = event-data() -> ("CtlRef"=w532:refnum<vi>, "Coords"=w541:T16, "Button"=w542:u16)  [unwired: 1 in, 3 out]
        n167 = case shown="3" w542 {
          tunnel: w541 -> [_ w552 _]
          tunnel: queue_action."GUI_plotSpectrumAutoScaleY" ("action") -> [w547 _ _]
          tunnel: [w547 w554 w557] -> w535
          tunnel: queue_action."GUI_plotSpectrumZoomMouse" ("action") -> [_ w554 _]
          tunnel: w532 -> [_ w553 _]
          tunnel: [0.0 ("X") w550 0.0 ("X")] -> w530
          tunnel: w529 -> [w545 w549 w555]
          tunnel: [w545 w548 w555] -> w528
          tunnel: queue_action."none" ("action") -> [_ _ w557]
          frame 2 {
          }
          frame 3 {
            n168 = invoke class="IntGraph (strict)" method="Map Coords To XY"(reference=w553, error in=w549, "Coords"=w552) -> (error out=w548:errorcluster, "XY"=w551:cluster{"X":dbl, "Y":dbl})  [unwired: 4 in, 5 out]
            n169 = Unbundle By Name(w551) -> ("X"=w550:dbl)
          }
          frame 1, Default {
          }
        }
        n170 = Bundle By Name(cluster=T12 {"action"=enum."none", "skip old"=FALSE, "force immidiate"=FALSE, "par"=0.0, "par 2"=0.0, "par 3"=0.0, "par 4"=0.0, "idx"=0, "idx 2"=0, "no duplicate"=FALSE} ("action data"), "action"=w535, "par"=w530) -> (w537:T12)
        n171 = Build Array(w537) -> (w538:T12[])
        n172 = call "action_define.vi"("action"=queue_action."ANALYSE_SPECTRUM", "action data"=w538, "error in (no error)"=w528, "skip old"=TRUE) -> ("action data out"=w531:T12[], "error out"=w543:errorcluster)  [unwired: 14 in]
      }
      event "Intensity Graph Interferogram": Mouse Up {
        n173 = event-data() -> ("CtlRef"=w566:refnum<vi>, "Coords"=w567:T16, "Button"=w559:u16)  [unwired: 1 in, 4 out]
        n174 = case shown="1, Default" w559 {
          tunnel: w567 -> [_ _ w586]
          tunnel: queue_action."GUI_plotInterferogramAutoScaleY" ("action") -> [w578 _ _]
          tunnel: [w578 w579 w588] -> w571
          tunnel: queue_action."GUI_plotInterferogramZoomMouse" ("action") -> [_ _ w588]
          tunnel: w566 -> [_ _ w587]
          tunnel: [0.0 ("X") 0.0 ("X") w584] -> w569
          tunnel: w565 -> [w576 w580 w583]
          tunnel: [w576 w580 w582] -> w568
          tunnel: queue_action."none" ("action") -> [_ w579 _]
          frame 2 {
          }
          frame 1, Default {
          }
          frame 3 {
            n175 = invoke class="IntGraph (strict)" method="Map Coords To XY"(reference=w587, error in=w583, "Coords"=w586) -> (error out=w582:errorcluster, "XY"=w585:cluster{"X":dbl, "Y":dbl})  [unwired: 4 in, 5 out]
            n176 = Unbundle By Name(w585) -> ("X"=w584:dbl)
          }
        }
        n177 = Bundle By Name(cluster=T12 {"action"=enum."none", "skip old"=FALSE, "force immidiate"=FALSE, "par"=0.0, "par 2"=0.0, "par 3"=0.0, "par 4"=0.0, "idx"=0, "idx 2"=0, "no duplicate"=FALSE} ("action data"), "action"=w571, "par"=w569) -> (w573:T12)
        n178 = Build Array(w573) -> (w574:T12[])
        n179 = call "action_define.vi"("action"=queue_action."ANALYSE_INTERFEROGRAM", "action data"=w574, "error in (no error)"=w568, "skip old"=TRUE) -> ("action data out"=w563:T12[], "error out"=w564:errorcluster)  [unwired: 14 in]
      }
      event "Intensity Graph Interferogram": Cursor Release {
        w593 = FALSE  # force immidiate
        w594 = TRUE  # skip old
        n180 = event-data() -> ()  [unwired: 1 in, 7 out]
        n181 = call "action_define.vi"("action"=queue_action."ANALYSE_INTERFEROGRAM", "error in (no error)"=w589, "skip old"=w594, "force immidiate"=w593) -> ("action data out"=w591:T12[], "error out"=w590:errorcluster)  [unwired: 14 in]
      }
      event "Intensity Graph spectrum": Cursor Release {
        w600 = FALSE  # force immidiate
        w601 = TRUE  # skip old
        n182 = event-data() -> ()  [unwired: 1 in, 7 out]
        n183 = call "action_define.vi"("action"=queue_action."ANALYSE_SPECTRUM", "error in (no error)"=w597, "skip old"=w601, "force immidiate"=w600) -> ("action data out"=w598:T12[], "error out"=w599:errorcluster)  [unwired: 14 in]
      }
      event Value Change {
        w605 = TRUE  # force immidiate
        w606 = TRUE  # skip old
        n184 = event-data() -> ("NewVal"=w603:T2)  [unwired: 1 in, 4 out]
        n185 = call "action_define.vi"("action"=queue_action."MODE_resolution set", "error in (no error)"=w608, "idx"=w603, "skip old"=w606, "force immidiate"=w605) -> ("action data out"=w609:T12[], "error out"=w610:errorcluster)  [unwired: 13 in]
      }
      event Value Change {
        w616 = TRUE  # force immidiate
        w617 = TRUE  # skip old
        n186 = event-data() -> ("NewVal"=w611:T3)  [unwired: 1 in, 4 out]
        n187 = call "action_define.vi"("action"=queue_action."MODE_sensitivity set", "error in (no error)"=w615, "idx"=w611, "skip old"=w617, "force immidiate"=w616) -> ("action data out"=w613:T12[], "error out"=w614:errorcluster)  [unwired: 13 in]
      }
      event Value Change {
        w619 = TRUE  # force immidiate
        w622 = TRUE  # skip old
        n188 = event-data() -> ("NewVal"=w621:T6)  [unwired: 1 in, 4 out]
        n189 = To Long Integer(number=w621) -> (32bit integer=w620:i32)
        n190 = call "action_define.vi"("action"=queue_action."ACQOPT_apodisation type set", "error in (no error)"=w624, "idx"=w620, "skip old"=w622, "force immidiate"=w619) -> ("action data out"=w626:T12[], "error out"=w627:errorcluster)  [unwired: 13 in]
      }
      event "average nr": Value Change {
        w628 = TRUE  # force immidiate
        w635 = TRUE  # skip old
        n191 = event-data() -> ("NewVal"=w630:u16)  [unwired: 1 in, 4 out]
        n192 = To Long Integer(number=w630) -> (32bit integer=w629:i32)
        n193 = call "action_define.vi"("action"=queue_action."ACQOPT_average spectrum set", "error in (no error)"=w633, "idx"=w629, "skip old"=w635, "force immidiate"=w628) -> ("action data out"=w631:T12[], "error out"=w634:errorcluster)  [unwired: 13 in]
      }
      event "rolling aver": Value Change {
        w637 = TRUE  # force immidiate
        w641 = TRUE  # skip old
        n194 = event-data() -> ("NewVal"=w640:bool)  [unwired: 1 in, 4 out]
        n195 = Boolean To (0,1)(Boolean=w640) -> (0, 1=w639:i16)
        n196 = To Long Integer(number=w639) -> (32bit integer=w638:i32)
        n197 = call "action_define.vi"("action"=queue_action."ACQOPT_rolling average set", "error in (no error)"=w645, "idx"=w638, "skip old"=w641, "force immidiate"=w637) -> ("action data out"=w644:T12[], "error out"=w643:errorcluster)  [unwired: 13 in]
      }
      event "acq delay (ms)": Value Change {
        w648 = TRUE  # force immidiate
        w651 = TRUE  # skip old
        n198 = event-data() -> ("NewVal"=w650:u32)  [unwired: 1 in, 4 out]
        n199 = To Long Integer(number=w650) -> (32bit integer=w649:i32)
        n200 = call "action_define.vi"("action"=queue_action."ACQOPT_acqIntervall_set", "error in (no error)"=w655, "idx"=w649, "skip old"=w651, "force immidiate"=w648) -> ("action data out"=w653:T12[], "error out"=w654:errorcluster)  [unwired: 13 in]
      }
      event Value Change {
        w661 = TRUE  # skip old
        n201 = event-data() -> ()  [unwired: 1 in, 5 out]
        n202 = call "action_define.vi"("action"=queue_action."MATH", "error in (no error)"=w660, "skip old"=w661) -> ("action data out"=w658:T12[], "error out"=w659:errorcluster)  [unwired: 15 in]
      }
      event Value Change {
        w667 = TRUE  # skip old
        n203 = event-data() -> ()  [unwired: 1 in, 5 out]
        n204 = call "action_define.vi"("action"=queue_action."ANALYSE_SPECTRUM", "error in (no error)"=w665, "skip old"=w667) -> ("action data out"=w663:T12[], "error out"=w664:errorcluster)  [unwired: 15 in]
      }
      event "pwr": Value Change {
        n205 = event-data() -> ("NewVal"=w678:bool)  [unwired: 1 in, 4 out]
        n206 = Unbundle By Name(w669) -> ("Power (Y unit)"=w668:refnum<vi>)
        n207 = case shown="False" w678 {
          tunnel: queue_action."ANALYSE_SPECTRUM" ("action") -> [_ w685]
          tunnel: [w683 w685] -> w673
          tunnel: queue_action."none" ("action") -> [w683 _]
          tunnel: w671 -> [w682 w684]
          tunnel: [w681 w684] -> w670
          tunnel: w668 -> [w680 _]
          frame False {
            n208 = property class="DigNum (strict)"(reference=w680, error in=w682, "Value"=-1.0) -> (error out=w681:errorcluster)  [unwired: 1 out]
          }
          frame True {
          }
        }
        n209 = call "action_define.vi"("action"=w673, "error in (no error)"=w670) -> ("action data out"=w676:T12[], "error out"=w677:errorcluster)  [unwired: 16 in]
      }
      event "Peak find": Value Change {
        n210 = event-data() -> ("NewVal"=w690:bool)  [unwired: 1 in, 4 out]
        n211 = Unbundle By Name(w688) -> ("Peak (X unit)"=w687:refnum<vi>)
        n212 = case shown="False" w690 {
          tunnel: queue_action."ANALYSE_SPECTRUM" ("action") -> [_ w703]
          tunnel: [w701 w703] -> w695
          tunnel: queue_action."none" ("action") -> [w701 _]
          tunnel: w689 -> [w700 w702]
          tunnel: w687 -> [w698 _]
          tunnel: [w699 w702] -> w686
          frame False {
            n213 = property class="DigNum (strict)"(reference=w698, error in=w700, "Value"=-1.0) -> (error out=w699:errorcluster)  [unwired: 1 out]
          }
          frame True {
          }
        }
        n214 = call "action_define.vi"("action"=w695, "error in (no error)"=w686) -> ("action data out"=w691:T12[], "error out"=w692:errorcluster)  [unwired: 16 in]
      }
      event "wmtr": Value Change {
        n215 = event-data() -> ("NewVal"=w706:bool)  [unwired: 1 in, 4 out]
        n216 = Unbundle By Name(w709) -> ("Wavemeter (/cm)"=w708:refnum<vi>)
        n217 = Boolean To (0,1)(Boolean=w706) -> (0, 1=w710:i16)
        n218 = call "action_define.vi"("action"=queue_action."ACQOPT_cycle counting set", "error in (no error)"=w712, "idx"=w710) -> ("action data out"=w705:T12[], "error out"=w707:errorcluster)  [unwired: 15 in]
        n219 = case shown="False" w706 {
          tunnel: w707 -> [w717 w718]
          tunnel: [w716 w718] -> w704
          tunnel: w708 -> [w714 _]
          frame False {
            n220 = property class="DigNum (strict)"(reference=w714, error in=w717, "Value"=-1.0) -> (error out=w716:errorcluster)  [unwired: 1 out]
          }
          frame True {
          }
        }
      }
      event "coh.l": Value Change {
        n221 = event-data() -> ("NewVal"=w726:bool)  [unwired: 1 in, 4 out]
        n222 = Unbundle By Name(w721) -> ("coherenceLength, (cm)"=w720:refnum<vi>)
        n223 = case shown="False" w726 {
          tunnel: queue_action."ANALYSE_INTERFEROGRAM" ("action") -> [_ w736]
          tunnel: [w734 w736] -> w729
          tunnel: queue_action."none" ("action") -> [w734 _]
          tunnel: w723 -> [w733 w735]
          tunnel: [w732 w735] -> w727
          tunnel: w720 -> [w730 _]
          frame False {
            n224 = property class="DigNum (strict)"(reference=w730, error in=w733, "Value"=-1.0) -> (error out=w732:errorcluster)  [unwired: 1 out]
          }
          frame True {
          }
        }
        n225 = call "action_define.vi"("action"=w729, "error in (no error)"=w727) -> ("action data out"=w722:T12[], "error out"=w719:errorcluster)  [unwired: 16 in]
      }
      event "auto": Value Change {
        n226 = event-data() -> ("NewVal"=w740:bool)  [unwired: 1 in, 5 out]
        n227 = Boolean To (0,1)(Boolean=w740) -> (0, 1=w739:i16)
        n228 = To Long Integer(number=w739) -> (32bit integer=w738:i32)
        n229 = call "action_define.vi"("action"=queue_action."ACQOPT_gainLevel auto set", "error in (no error)"=w743, "idx"=w738) -> ("action data out"=w741:T12[], "error out"=w742:errorcluster)  [unwired: 15 in]
      }
      event "gain": Value Change {
        n230 = event-data() -> ("NewVal"=w752:u16)  [unwired: 1 in, 5 out]
        n231 = Unbundle By Name(w756) -> ("auto"=w755:refnum<vi>)
        n232 = property class="Bool (strict)"(reference=w755) -> ("Value"=w750:bool)  [unwired: 1 in, 2 out]
        n233 = To Long Integer(number=w752) -> (32bit integer=w751:i32)
        n234 = Select(t=queue_action."none" ("action"), s=w750, f=queue_action."ACQOPT_gainLevel set" ("action")) -> (s? t:f=w747:T13)
        n235 = call "action_define.vi"("action"=w747, "error in (no error)"=w754, "idx"=w751) -> ("action data out"=w746:T12[], "error out"=w753:errorcluster)  [unwired: 15 in]
      }
      event Value Change {
        n236 = event-data() -> ("NewVal"=w761:T1)  [unwired: 1 in, 5 out]
        n237 = To Long Integer(number=w761) -> (32bit integer=w760:i32)
        n238 = call "action_define.vi"("action"=queue_action."MODE_PDTemperature set", "error in (no error)"=w764, "idx"=w760, "skip old"=TRUE) -> ("action data out"=w759:T12[], "error out"=w763:errorcluster)  [unwired: 14 in]
      }
      event "exit butt": Value Change {
        n239 = event-data() -> ("NewVal"=w768:bool)  [unwired: 1 in, 4 out]
        n240 = case shown="True" w768 {
          tunnel: queue_action."stop" ("action") -> [_ w774]
          tunnel: [w773 w774] -> w766
          tunnel: queue_action."none" ("action") -> [w773 _]
          frame False {
          }
          frame True {
          }
        }
        n241 = call "action_define.vi"("action"=w766, "error in (no error)"=w772) -> ("action data out"=w770:T12[], "error out"=w771:errorcluster)  [unwired: 16 in]
        n242 = stacked-sequence {
          tunnel: ["exit butt"] -> _
          tunnel: w771 -> [_]
          frame #0 {
          }
        }
      }
    }
    n243 = call "action_set.vi"("reference"=w426, "action data"=w423, "error in (no error)"=w427) -> ("duplicate reference"=w424:refnum<class "OSA.lvclass">, "error out"=w425:errorcluster)  [unwired: 15 in]
    n244 = call "Stop.vi"("reference"=w424, "error in (no error)"=w425) -> ("reference"=w430:refnum<class "OSA.lvclass">, "Stop"=w429:bool, "error out"=w432:errorcluster)  [unwired: 15 in]
  }
  n245 = Merge Errors(w47, w46, w45) -> (w26:errorcluster)
  n246 = call "close.vi"("reference"=w25, "error in (no error)"=w26) -> ("error out"=w48:errorcluster)  [unwired: 17 in]
  n247 = call <vilib>:"Simple Error Handler.vi"("error in (no error)"=w48) -> ()  [unwired: 4 in, 5 out]
